vi "ABR-Create Stimulus.vi"(0 "Stimulus":T3={"Ear"=enum."Left", "Start (dB)"=20, "Waveform"=enum."TONE PIP", "Stop (dB)"=80, "Frequency (kHz)"=16.0, "Step (dB)"=5, "Rep rate (/sec)"=30.0, "Alternate Polarity"=FALSE} {"Frequency (kHz)" format="%.2f"; "Start (dB)" step=5}, 5 "Runtime":T1, 9 "Hidden":T2={"AI Samp Rate Hz"=25000.0, "AO Samp Rate Hz"=100000.0, "Duration (ms)"=5.0, "Ramp (ms)"=0.5, "Click width (us)"=0.0, "ITI"=enum."Rate", "Save raw"=FALSE}, 11 "error in (no error)":errorcluster) -> (8 "stimulus":dbl[][](array[numeric]), 15 "error out":errorcluster)   [LabVIEW 2020]
uses:
  PXI DAQ VIs/DAQ Engine VIs/PXI Globals.vi
  Signal Synthesis VIs/Waveform VIs/Pulse Train VIs/Pulse Polarity.ctl
  Signal Synthesis VIs/Waveform VIs/Pulse Train VIs/Pulse Train Params.ctl
  Signal Synthesis VIs/Waveform VIs/Pulse Train VIs/PT-Continuous State.ctl
  Typedefs/ABR-Stimulus.ctl
  TypeDefs/ABR-Hidden Params.ctl
  Typedefs/ABR-Runtime Data.ctl
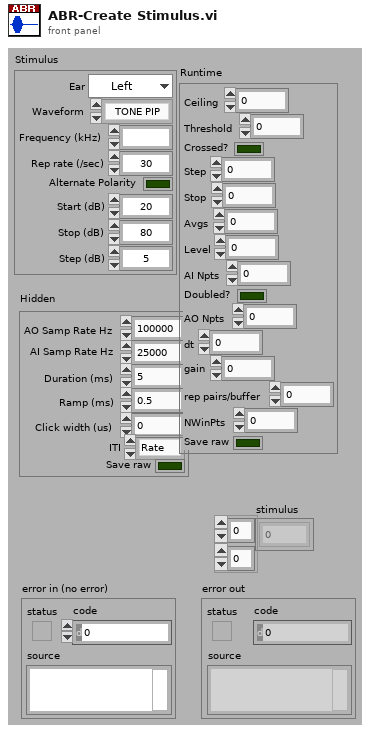
[diagram p1: front panel]
types:
  T1 = typedef "ABR-Runtime Data.ctl" = cluster{"Ceiling":dbl, "Threshold":dbl, "Crossed?":bool, "Step":dbl, "Stop":i32, "Avgs":i32, "Level":dbl, "AI Npts":i32, "Doubled?":bool, "AO Npts":i32, "dt":dbl, "gain":dbl, "rep pairs/buffer":i32, "NWinPts":i32, "Save raw":bool}
  T2 = typedef "ABR-Hidden Params.ctl" = cluster{"AI Samp Rate Hz":dbl, "AO Samp Rate Hz":dbl, "Duration (ms)":dbl, "Ramp (ms)":dbl, "Click width (us)":dbl, "ITI":enum16{"Rate", "Interval"}, "Save raw":bool}
  T3 = typedef "ABR-Stimulus.ctl" = cluster{"Ear":enum16{"Right", "Left", "Bone"}, "Start (dB)":i32, "Waveform":enum16{"TONE PIP", "CLICK"}, "Stop (dB)":i32, "Frequency (kHz)":ext, "Step (dB)":i32, "Rep rate (/sec)":dbl, "Alternate Polarity":bool}
  T4 = cluster{"Active":bool, "Delay (ms)":dbl, "Width (ms)":dbl, "Ramp (ms)":dbl}
  T5 = typedef "Pulse Train Params.ctl" = cluster{"Pulse width (us)":dbl, "Pulse rate (Hz)":dbl, "Gap (ms)":dbl, "Polarity":T6, "PT State":T7, "Asynch":bool}
  T6 = typedef "Pulse Polarity.ctl" = enum16{"POS", "NEG", "POS-NEG", "NEG-POS"}
  T7 = typedef "PT-Continuous State.ctl" = cluster{"Template":dbl[], "Nperiod":i32, "Index":i32, "Pulse Rate (Hz)":dbl, "Phase (cycles)":dbl, "Noff":i32}
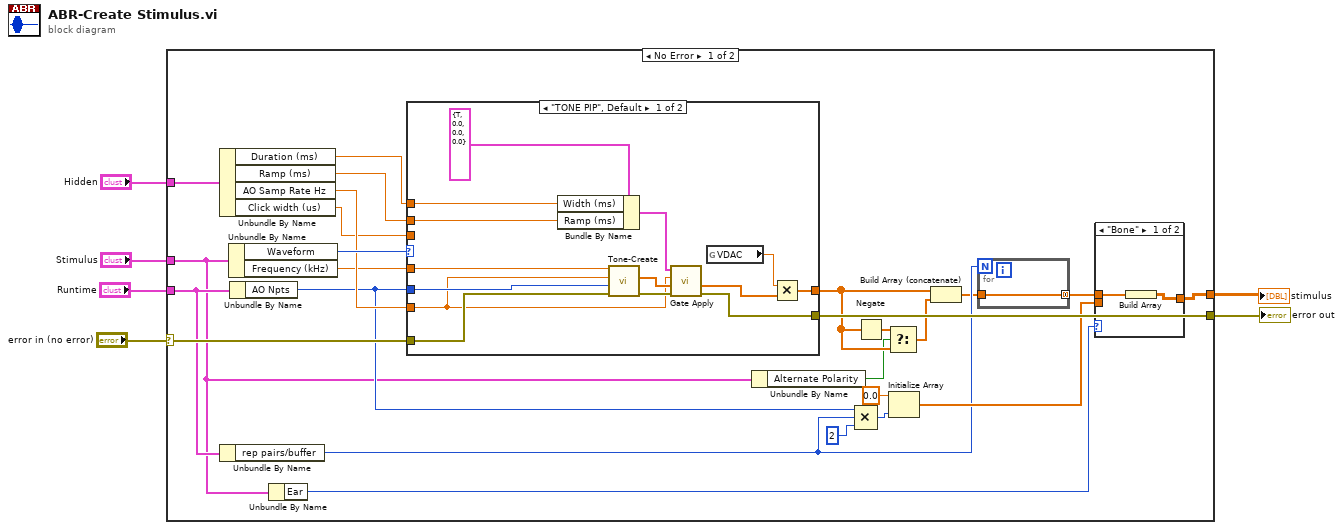
[diagram p0: block diagram]
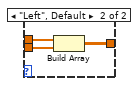
[diagram p2: hidden frame]
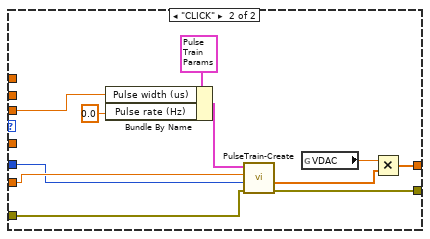
[diagram p3: hidden frame]
diagram:
  n1 = case shown="No Error" "error in (no error)" {
    selector: "error in (no error)" -> [w20 w63]
    tunnel: [w31 w63] -> w6
    tunnel: "Stimulus" -> [w8 _]
    tunnel: [w25 _] -> w4
    tunnel: "Hidden" -> [w24 _]
    tunnel: "Runtime" -> [w12 _]
    frame No Error {
      n2 = Unbundle By Name(w24) -> ("Duration (ms)"=w23:dbl, "Ramp (ms)"=w22:dbl, "AO Samp Rate Hz"=w21:dbl, "Click width (us)"=w19:dbl)
      n3 = Unbundle By Name(w12) -> ("rep pairs/buffer"=w11:i32)
      n4 = Unbundle By Name(w8) -> ("Waveform"=w26:enum16{"TONE PIP", "CLICK"}, "Frequency (kHz)"=w14:ext)
      n5 = Unbundle By Name(w12) -> ("AO Npts"=w13:i32)
      n6 = Unbundle By Name(w8) -> ("Ear"=w7:enum16{"Right", "Left", "Bone"})
      n7 = case shown="\"TONE PIP\", Default" w26 {
        tunnel: w20 -> [w51 w60]
        tunnel: w23 -> [w50 _]
        tunnel: w22 -> [w49 _]
        tunnel: [w45 w61] -> w31
        tunnel: [w44 w55] -> w29
        tunnel: w21 -> [w39 w58]
        tunnel: w13 -> [w42 w57]
        tunnel: w14 -> [w38 _]
        tunnel: w19 -> [_ w52]
        frame "TONE PIP", Default {
          n8 = Bundle By Name(cluster=T4 {"Active"=TRUE, "Delay (ms)"=0.0, "Width (ms)"=0.0, "Ramp (ms)"=0.0} ("Gate Control"), "Width (ms)"=w50, "Ramp (ms)"=w49) -> (w40:T4)
          n9 = call "Tone-Create.vi"("error in (no error)"=w51, "Npts"=w42, "Sampling Rate (Hz)"=w39, "Frequency (kHz)"=w38) -> ("error out"=w48:errorcluster, "Waveform"=w47:dbl[])  [unwired: 6 in]
          n10 = call "Gate Apply.vi"("error in (no error)"=w48, "Waveform in"=w47, "Sampling Rate (Hz)"=w39, "Gate Control"=w40) -> ("error out"=w45:errorcluster, "Gated waveform"=w46:dbl[])  [unwired: 6 in]
          n11 = global read "PXI Globals.vi" "VDAC"() -> (w43:dbl)
          n12 = Multiply(x=w43, y=w46) -> (x*y=w44:dbl[])
        }
        frame "CLICK" {
          n13 = Bundle By Name(cluster=T5 {"Pulse width (us)"=0.0, "Pulse rate (Hz)"=0.0, "Gap (ms)"=0.0, "Polarity"=enum."POS", "PT State"={"Template"=[], "Nperiod"=0, "Index"=0, "Pulse Rate (Hz)"=0.0, "Phase (cycles)"=0.0, "Noff"=0}, "Asynch"=FALSE} ("Pulse Train Params"), "Pulse width (us)"=w52, "Pulse rate (Hz)"=0.0) -> (w59:T5)
          n14 = call "PulseTrain-Create.vi"("error in (no error)"=w60, "Npts"=w57, "Sampling Rate (Hz)"=w58, "Pulse Train Params"=w59) -> ("error out"=w61:errorcluster, "Waveform"=w54:dbl[])  [unwired: 4 in, 2 out]
          n15 = global read "PXI Globals.vi" "VDAC"() -> (w53:dbl)
          n16 = Multiply(x=w53, y=w54) -> (x*y=w55:dbl[])
        }
      }
      n17 = Unbundle By Name(w8) -> ("Alternate Polarity"=w27:bool)
      n18 = Compound Arithmetic op=MULTIPLY(w13, w11, 2 ("y")) -> (w17:i32)
      n19 = Negate(x=w29) -> (-x=w28:dbl[])
      n20 = Select(t=w28, s=w27, f=w29) -> (s? t:f=w30:dbl[])
      n21 = Initialize Array(0.0 ("element"), w17) -> (w16:dbl[])
      n22 = Build Array (concatenate)(w29, w30) -> (w10:dbl[])
      n23 = for {
        N: w11 -> [_]
        tunnel: w10 -> [w37]
        tunnel: [w37] -> w9 mode=concatenating
      }
      n24 = case shown="\"Bone\"" w7 {
        tunnel: [w32 w36] -> w25
        tunnel: w16 -> [_ w35]
        tunnel: w9 -> [w33 w34]
        frame "Bone" {
          n25 = Build Array(w33) -> (w32:dbl[][])
        }
        frame "Left", Default {
          n26 = Build Array(w34, w35) -> (w36:dbl[][])
        }
      }
    }
    frame Error {
    }
  }
  "error out" <- w6
  "stimulus" <- w4
